vi "streaming_demo.vi"() -> ()   [LabVIEW 2012]
uses:
  <vilib>/measure/NI_MABase.lvlib
panel:
  out "error out":errorcluster
  in  "error in (no error)":errorcluster
  in  "Offset_I":dbl=77.0
  in  "Coeff_I":dbl=42.391
  in  "Offset_U":dbl=6.5
  in  "Coeff_U":dbl=2.55
  out "Time_indicator":dbl format="%.1f"
  out "Ток":dbl[](graph)
  out "Напряжение":dbl[](graph)
  in  "Стоп":bool
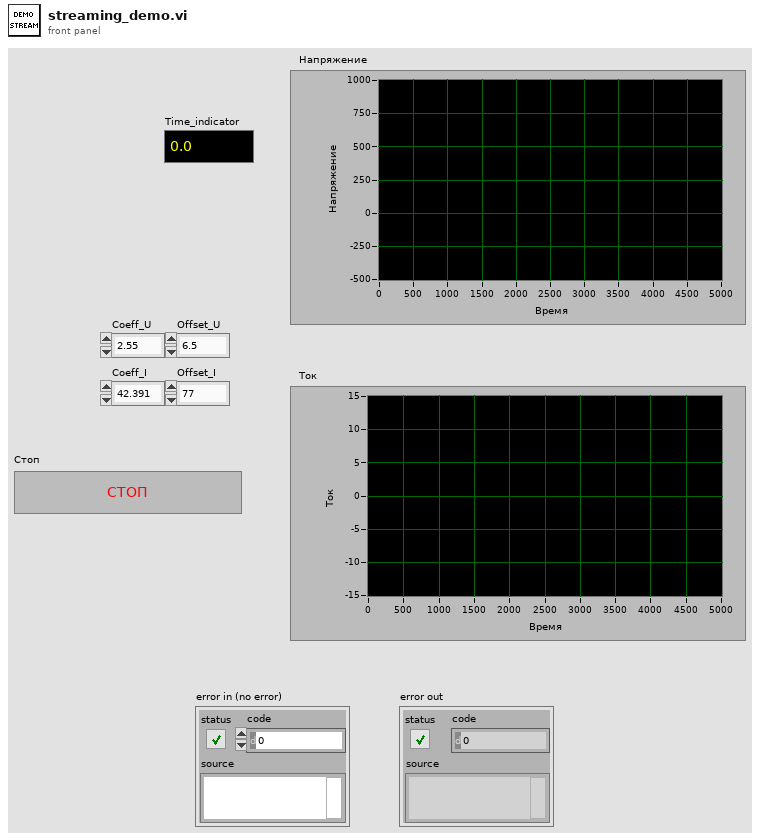
[diagram p1: front panel]
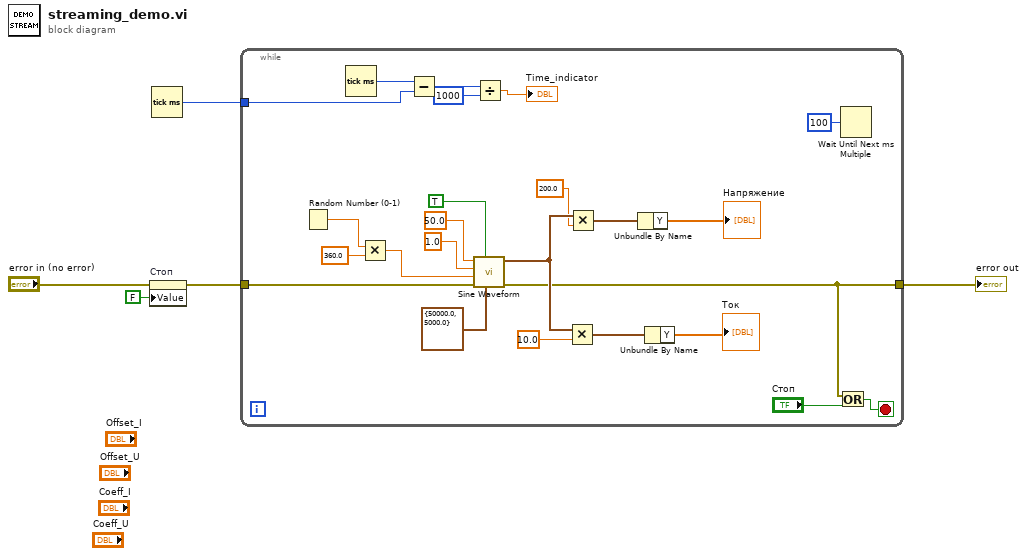
[diagram p0: block diagram]
diagram:
  n1 = property on="Стоп" class="Bool (strict)"(error in="error in (no error)", "Value"=FALSE ("Стоп")) -> (error out=w5:errorcluster)  [unwired: 1 in, 1 out]
  n2 = Tick Count (ms)() -> (millisecond timer value=w2:u32)
  n3 = while {
    tunnel: w5 -> [w19]
    tunnel: [w18] -> w3
    tunnel: w2 -> [w13]
    stop <- w16 stop-if-true
    n4 = Random Number (0-1)() -> (number: 0 to 1=w26:dbl)
    n5 = Tick Count (ms)() -> (millisecond timer value=w14:u32)
    n6 = Multiply(x=w26, y=360.0) -> (x*y=w28:dbl)
    n7 = Subtract(x=w14, y=w13) -> (x-y=w12:u32)
    n8 = call <vilib>:"Sine Waveform.vi"("sampling info"=cluster{"Fs":dbl, "#s":dbl} {"Fs"=50000.0, "#s"=5000.0}, "reset signal"=TRUE, "error in (no error)"=w19, "phase"=w28, "amplitude"=1.0, "frequency"=50.0) -> ("error out"=w18:errorcluster, "signal out"=w25:waveform(dbl))  [unwired: 4 in]
    n9 = Divide(x=w12, y=u32 1000) -> (x/y=→"Time_indicator":dbl)
    n10 = Multiply(x=w25, y=10.0) -> (x*y=w7:waveform(dbl))
    n11 = Multiply(x=w25, y=200.0) -> (x*y=w9:waveform(dbl))
    n12 = Unbundle By Name(w9) -> ("Y"=→"Напряжение":dbl[])
    n13 = Unbundle By Name(w7) -> ("Y"=→"Ток":dbl[])
    n14 = Or(x=w18, y="Стоп") -> (x .or. y?=w16:bool)
    n15 = Wait Until Next ms Multiple(millisecond multiple=u32 100) -> ()  [unwired: 1 out]
  }
  "error out" <- w3
